vi "Recurse Path 2.vi"(8 "Double Visit":bool, 9 "Next Cave":i32, 10 "Parent Path":T1, 11 "Cave System In":T2) -> (2 "Found Paths":T1[](array[typedef]))   [LabVIEW 2020]
uses:
  Cave System.ctl
  Cave.ctl
  Path.ctl
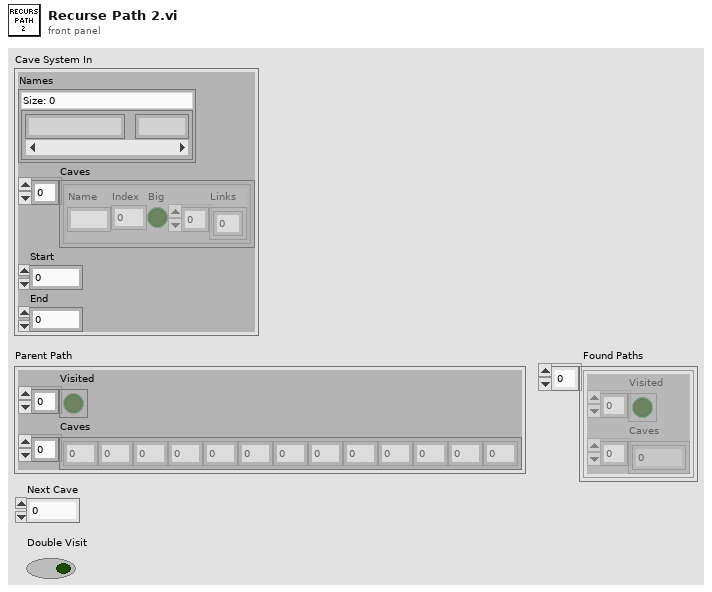
[diagram p1: front panel]
types:
  T1 = typedef "Path.ctl" = cluster{"Visited":bool[], "Caves":i32[]}
  T2 = typedef "Cave System.ctl" = cluster{"Names":map{string, i32}, "Caves":T3[], "Start":i32, "End":i32}
  T3 = typedef "Cave.ctl" = cluster{"Name":string, "Index":i32, "Big":bool, "Links":i32[]}
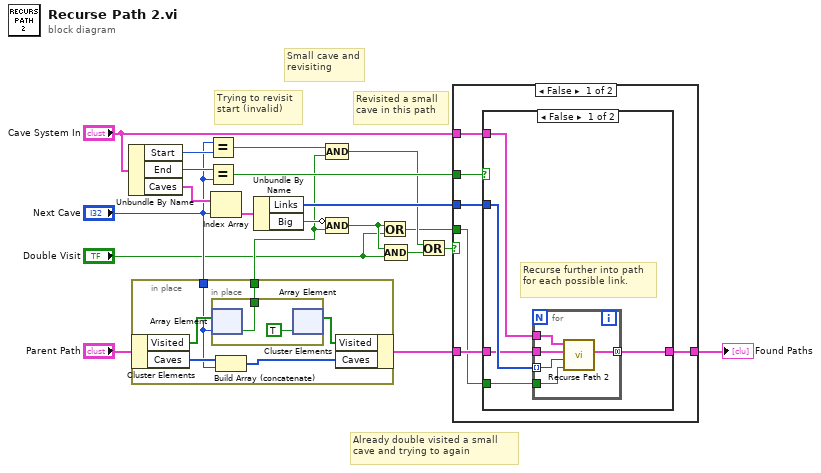
[diagram p0: block diagram]
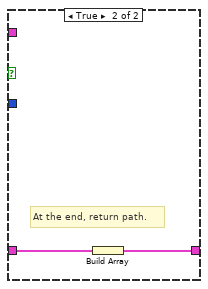
[diagram p2: hidden frame]
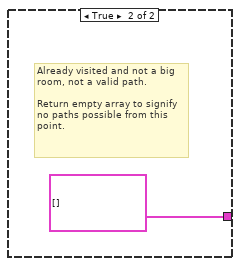
[diagram p3: hidden frame]
diagram:
  # "Already double visited a small cave and trying to again"
  # "Revisited a small cave in this path"
  # "Small cave and revisiting"
  # "Trying to revisit start (invalid)"
  n1 = Unbundle By Name("Cave System In") -> ("Start"=w9:i32, "End"=w13:i32, "Caves"=w19:T3[])
  n2 = in-place {
    in-place-border: [w25] -> w4
    in-place-border: "Next Cave" -> [w23]
    n3 = in-place-cluster #1("Parent Path") -> ("Visited"=w26:bool[], "Caves"=w24:i32[])
    n4 = in-place {
      in-place-border: [w28] -> w25
      n5 = in-place-array #2(w26, w23) -> (w28:bool)
      n6 = in-place-array #2(TRUE ("element")) -> (w22:bool[])  [unwired: 1 out]
    }
    n7 = Build Array (concatenate)(w24, w23) -> (w21:i32[])
    n8 = in-place-cluster #1("Visited"=w22, "Caves"=w21) -> (w16:T1)
  }
  n9 = Equal?(x="Next Cave", y=w9) -> (x = y?=w1:bool)
  n10 = Equal?(x=w13, y="Next Cave") -> (x = y?=w7:bool)
  n11 = Index Array(array=w19, index="Next Cave") -> (element=w18:T3)
  n12 = Unbundle By Name(w18) -> ("Links"=w15:i32[], "Big"=w17:bool)
  n13 = Compound Arithmetic op=AND(w1, w4) -> (w5:bool)
  n14 = Compound Arithmetic op=AND(invert w17, w4) -> (w11:bool)
  n15 = Or(x=w11, y="Double Visit") -> (x .or. y?=w3:bool)
  n16 = Compound Arithmetic op=AND(w11, "Double Visit") -> (w10:bool)
  n17 = Or(x=w5, y=w10) -> (x .or. y?=w6:bool)
  n18 = case shown="False" w6 {
    tunnel: w16 -> [w33 _]
    tunnel: w15 -> [w31 _]
    tunnel: [w32 T1[] [] ("Found Paths")] -> w14
    tunnel: w7 -> [w34 _]
    tunnel: "Cave System In" -> [w30 _]
    tunnel: w3 -> [w29 _]
    frame False {
      n19 = case shown="False" w34 {
        tunnel: w33 -> [w38 w46]
        tunnel: [w37 w45] -> w32
        tunnel: w31 -> [w39 _]
        tunnel: w30 -> [w36 _]
        tunnel: w29 -> [w35 _]
        frame False {
          # "Recurse further into path for each possible link."
          n20 = for {
            tunnel: w39 -> [w44] mode=indexing
            tunnel: w38 -> [w43]
            tunnel: [w42] -> w37 mode=concatenating
            tunnel: w36 -> [w41]
            tunnel: w35 -> [w40]
            n21 = call "Recurse Path 2.vi"("Double Visit"=w40, "Next Cave"=w44, "Parent Path"=w43, "Cave System In"=w41) -> ("Found Paths"=w42:T1[])  [unwired: 7 in]
          }
        }
        frame True {
          # "At the end, return path."
          n22 = Build Array(w46) -> (w45:T1[])
        }
      }
    }
    frame True {
      # "Already visited and not a big room, not a valid path.\n\nReturn empty array to signify no paths possible from this point."
    }
  }
  "Found Paths" <- w14
